vi "Process.vi"(8 "error in":errorcluster, 11 "DisplayWaveforms":refnum<class "DisplayWaveforms.lvclass">) -> (0 "error out":errorcluster, 3 "DisplayWaveforms out":refnum<class "DisplayWaveforms.lvclass">)   [LabVIEW 2020, in "DisplayWaveform.lvlib" / "DisplayWaveforms.lvclass"]
doc: "Displays all the waveforms using charts."
uses:
  DisplayWaveforms.lvclass
  C:/Program Files (x86)/National Instruments/LabVIEW 2020/vi.lib/JKI/JKI SMO/SMO/SMO.lvclass
  C:/Program Files (x86)/National Instruments/LabVIEW 2020/vi.lib/JKI/JKI SMO/SMO.UI/SMO.UI.lvclass
  <vilib>/JKI/JKI SMO/SMO/Typedefs/Parent Call--Enum.ctl
  PumpMeas/TypeDefs/ChartParamsCluster.ctl
  PumpMeas/TypeDefs/NI9205offset.ctl
  PumpMeas/TypeDefs/NI9205multiplier.ctl
  PumpMeas/TypeDefs/NI9208offset.ctl
  PumpMeas/TypeDefs/NI9208multiplier.ctl
  DisplayWaveforms.lvclass/DisplayWaveforms.ctl
  <vilib>/JKI/JKI SMO/SMO.UI/SMO.UI.lvclass
  <vilib>/JKI/JKI SMO/SMO/SMO.lvclass
panel:
  out "<TBD>":dbl[][](graph)
  out "<TBD>":dbl[][](graph)
  out "NI9208 Signals":dbl[][](graph)
  out "NI 9205 Signals":dbl[][](graph)
  out "NI9205 Signals":dbl[][](graph)
  in  "------------- Registered Events -------------":bool
  in  "------------- Public API -------------":bool
  # "For instructions on how to use the JKI State Machine Objects, examples and video tutorials, visit:\nhttp://jki.net/state-machine-objects/\n\nJKI State Machine Objects™\nhttp://jki.net/state-machine-objects/\nCopyright (C) 2005-2015, JKI <info@jki.net>\nALL RIGHTS RESERVED"
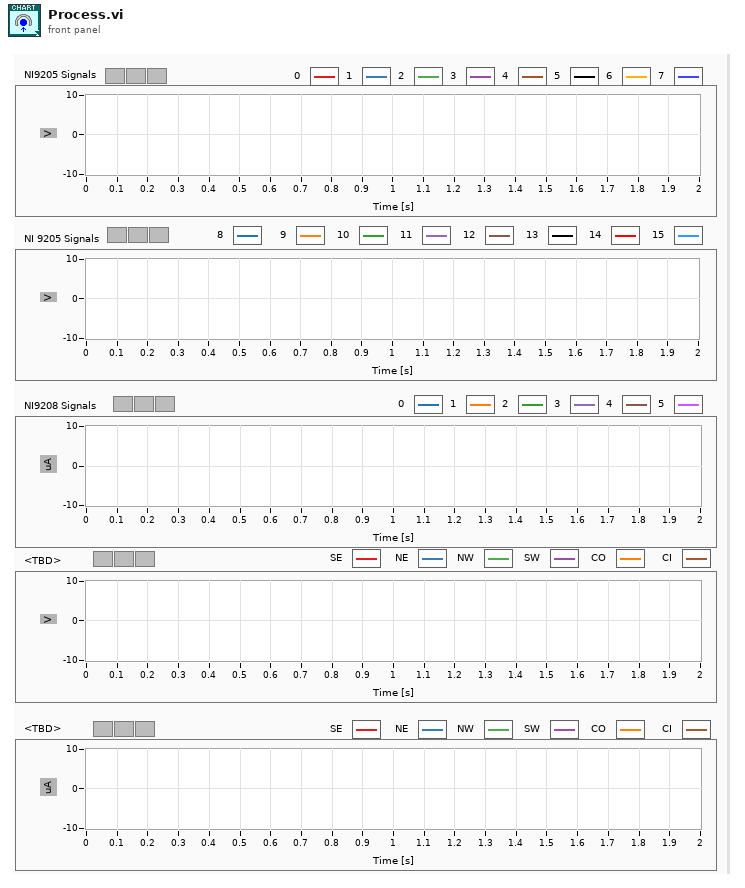
[diagram p1: front panel]
types:
  T1 = typedef "SMO.lvclass/Parent Call--Enum.ctl" = enum16{"Allows parent to run", "Does not request parent to run"}
  T2 = enum32{"invalid app kind", "Development System", "Run Time System", "Student Edition", "Embedded LabVIEW", "Evaluation", "Custom"}
  T3 = enum32{"Invalid", "Standard", "Closed", "Hidden", "Minimized", "Maximized"}
  T4 = typedef "ChartParamsCluster.ctl" = cluster{"Chart ScaleMultipliers":cluster{"WF Xscale Multiplier":dbl, "WF Yscale Multiplier":dbl[]}, "NI9205 Offset":T5, "NI9205 Multipliers":T6, "NI9208 Offset":T7, "NI9208 Multiplier":T8}
  T5 = typedef "NI9205offset.ctl" = cluster{"NI9205 Offset":dbl[]}
  T6 = typedef "NI9205multiplier.ctl" = cluster{"NI9205 Multiplier":dbl[]}
  T7 = typedef "NI9208offset.ctl" = cluster{"NI9208 Offset":dbl[]}
  T8 = typedef "NI9208multiplier.ctl" = cluster{"NI9208 Multiplier":dbl[]}
  T9 = cluster{"Core":cluster{"Current VI Reference":refnum<vi>, "Close Panel on Exit?":bool, "error":errorcluster}, "Self Reference":refnum<class "DisplayWaveforms.lvclass">, "bool":bool, "update chart?":bool, "ChartParams":T4, "Export Folder Path":path}
  T10 = cluster{"Current VI Reference":refnum<vi>, "Close Panel on Exit?":bool, "error":errorcluster}
  T11 = typedef "SMO.lvclass/Protected Events.ctl" = cluster{"StopProcesses":refnum<user-event>, "AbortProcesses":refnum<user-event>, "Config Changed":refnum<user-event>, "Dependency":refnum<user-event>}
  T12 = typedef "DisplayWaveform.lvlib/DisplayWaveforms.lvclass/ProtectedEvents--Cluster.ctl" = cluster{"Clear Chart":refnum<user-event>, "Pause Chart":refnum<user-event>, "Update Chart":refnum<user-event>, "Export Chart":refnum<user-event>, "Set ChartParams":refnum<user-event>}
  T13 = typedef "DisplayWaveform.lvlib/DisplayWaveforms.lvclass/Dependencies--Cluster.ctl" = cluster{"New Value":refnum<user-event>}
  T14 = typedef "imagedata.ctl" = cluster{"image type":i32, "image depth":i32, "image":u8[], "mask":u8[], "colors":u32[], "Rectangle":cluster{"left":i16, "top":i16, "right":i16, "bottom":i16}}
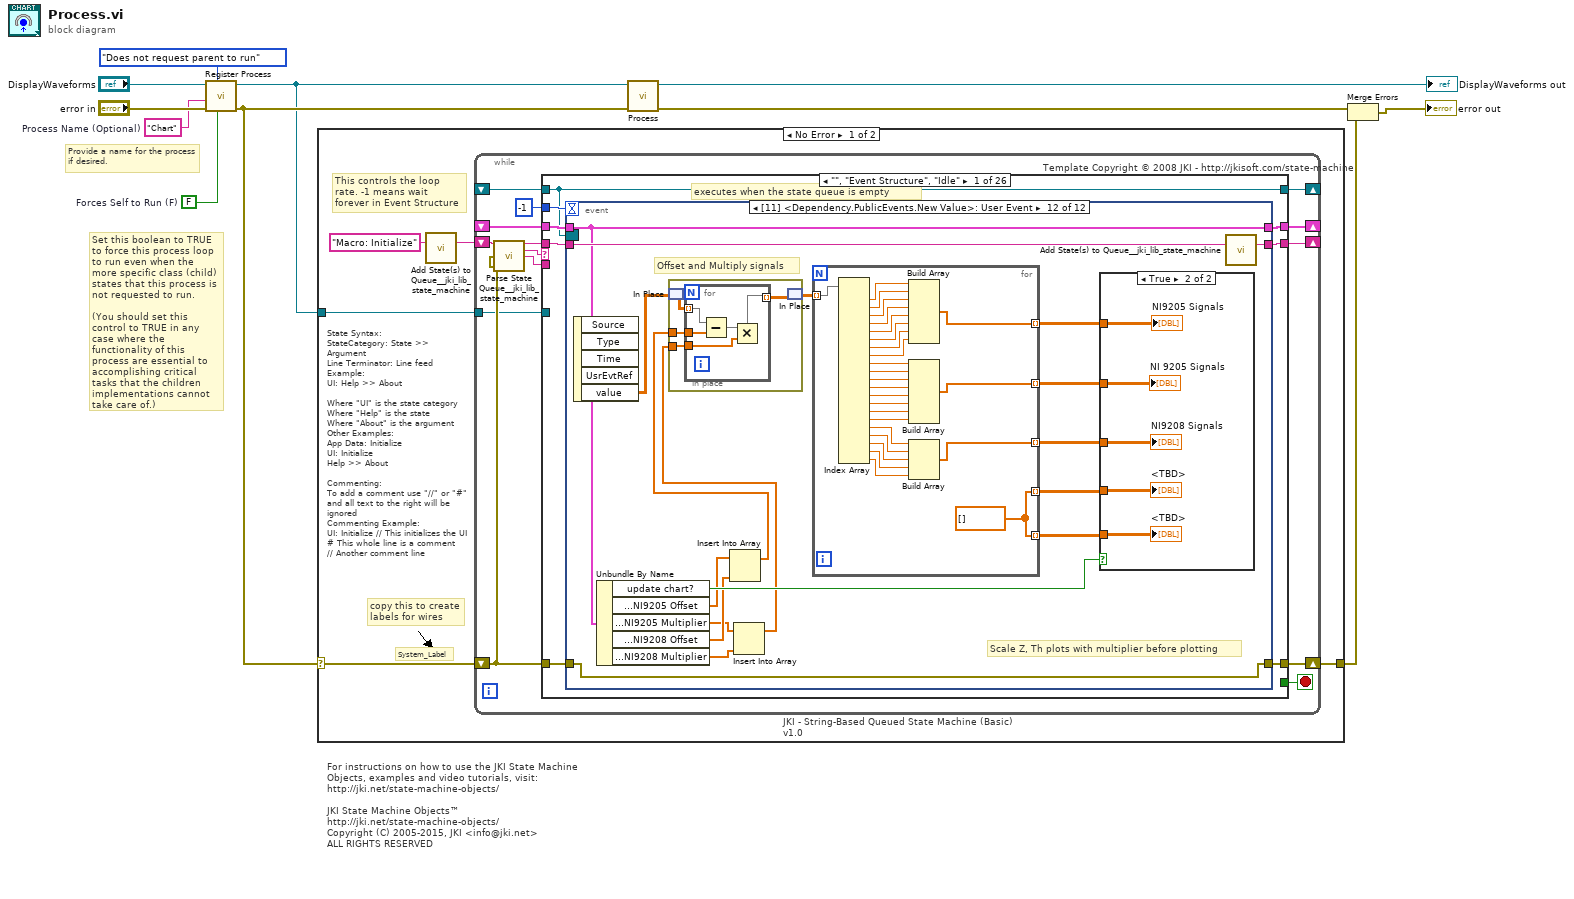
[diagram p0: block diagram]
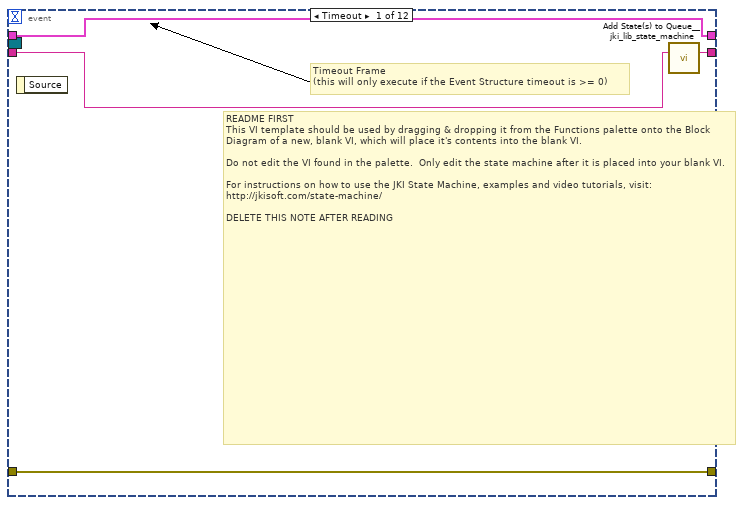
[diagram p2: hidden frame]
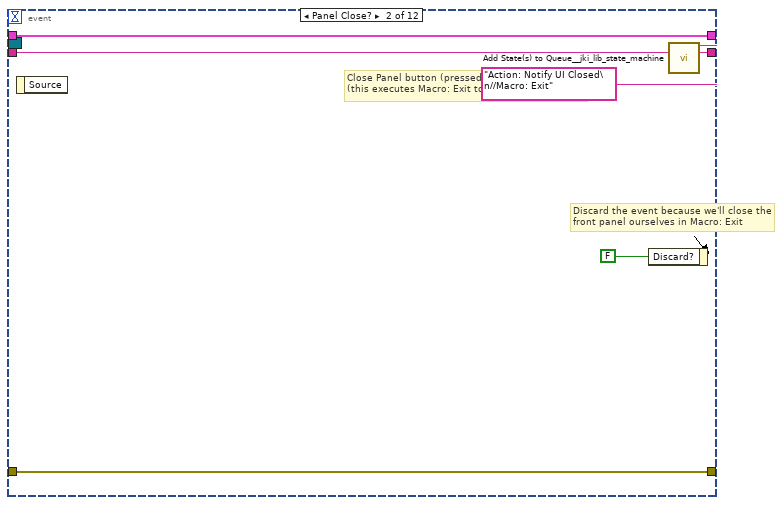
[diagram p3: hidden frame]
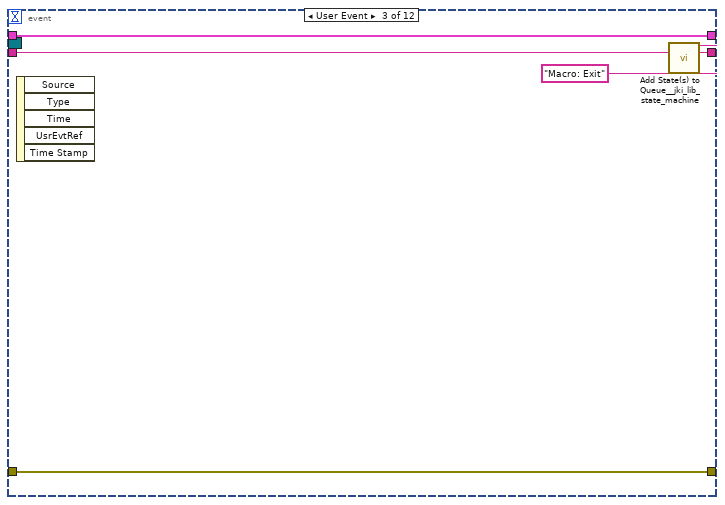
[diagram p4: hidden frame]
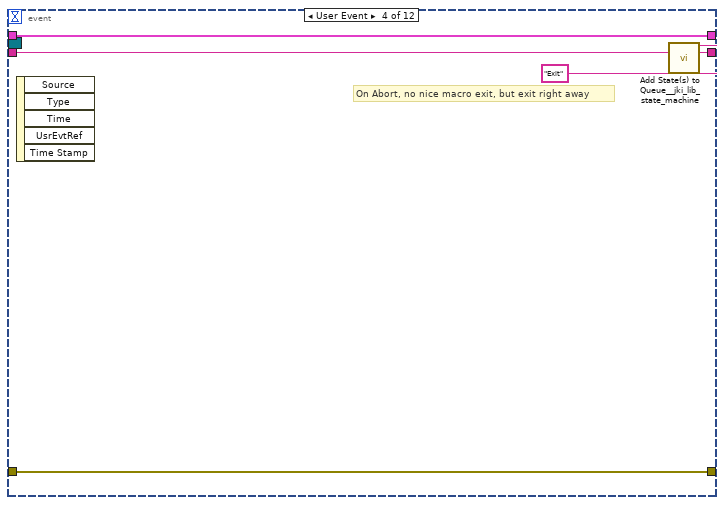
[diagram p5: hidden frame]
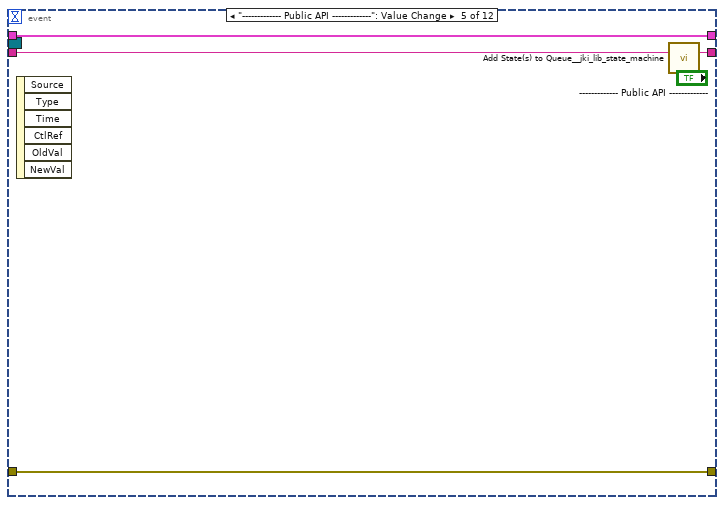
[diagram p6: hidden frame]
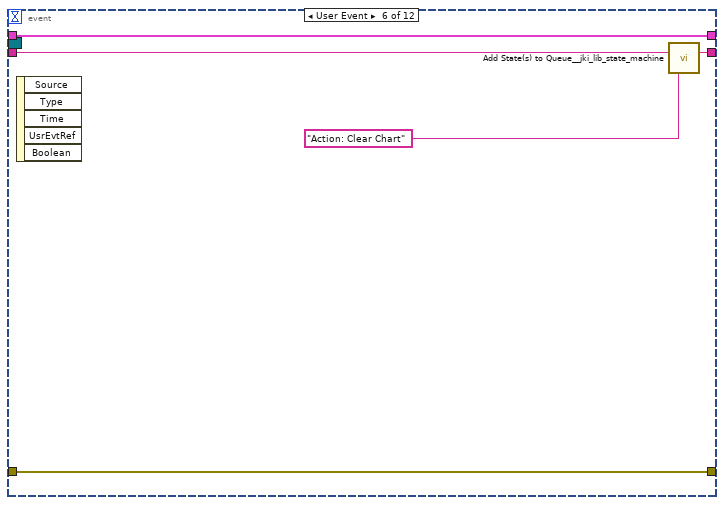
[diagram p7: hidden frame]
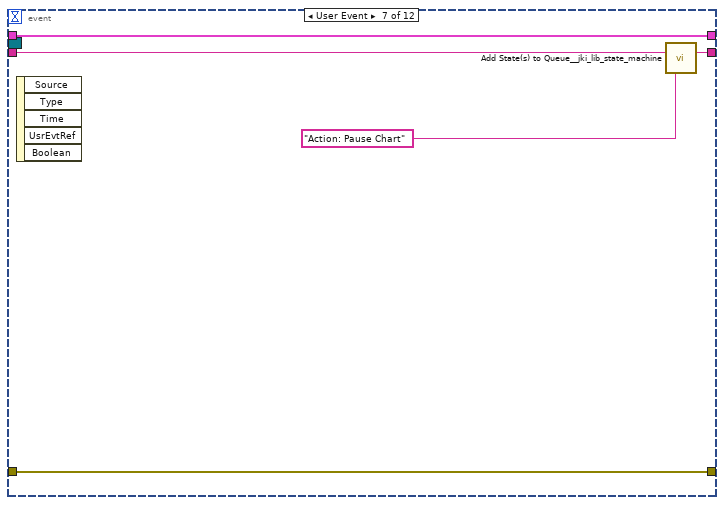
[diagram p8: hidden frame]
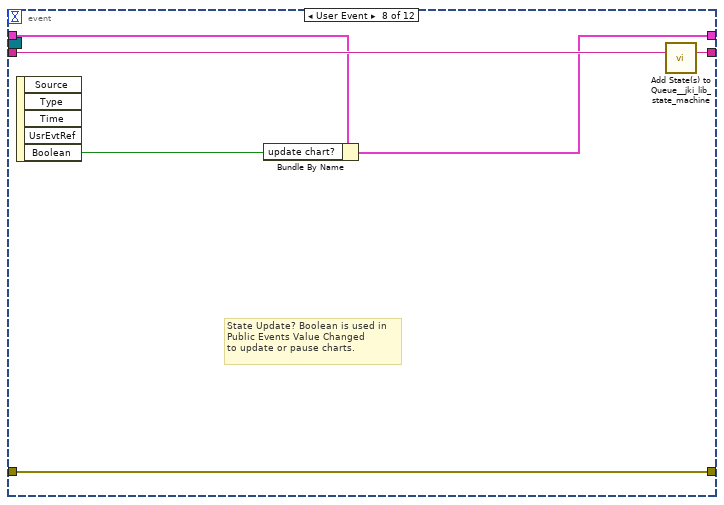
[diagram p9: hidden frame]
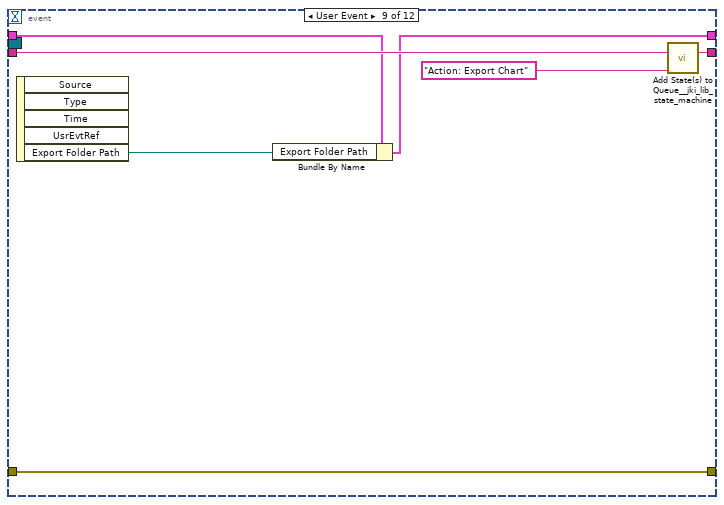
[diagram p10: hidden frame]
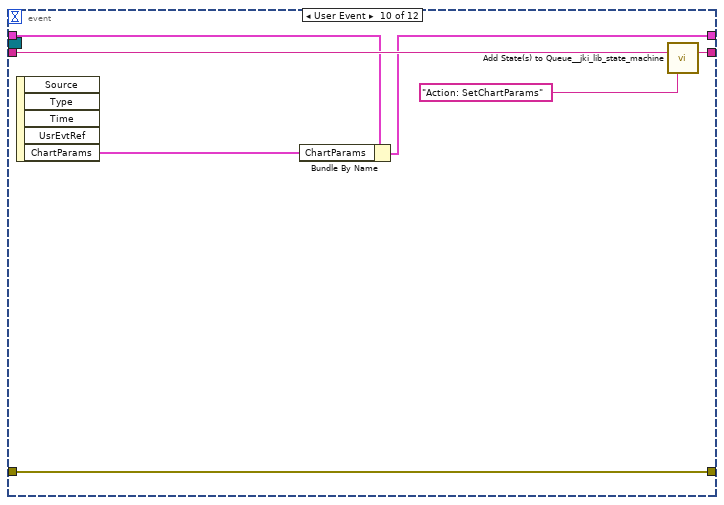
[diagram p11: hidden frame]
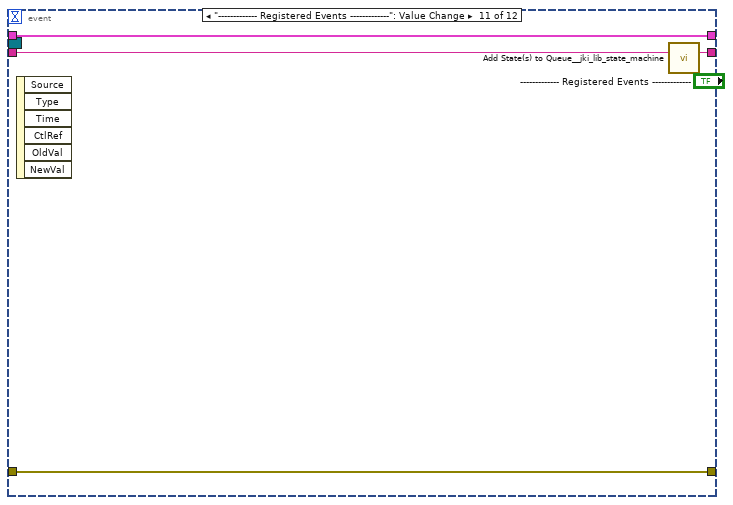
[diagram p12: hidden frame]
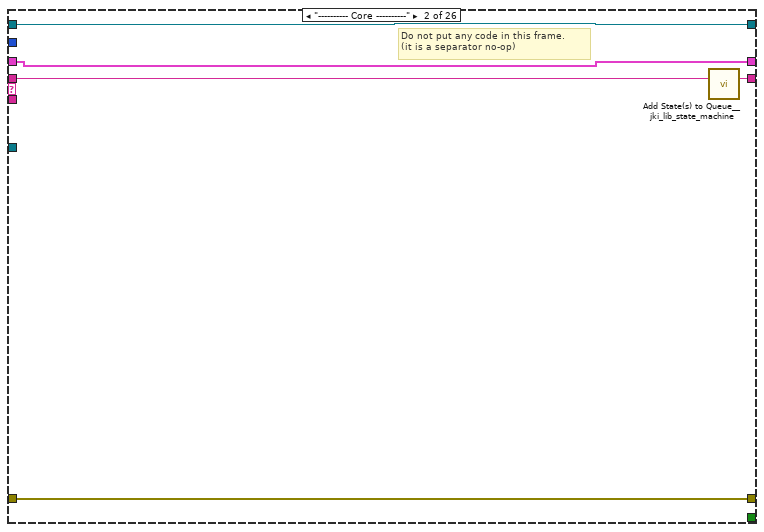
[diagram p14: hidden frame]
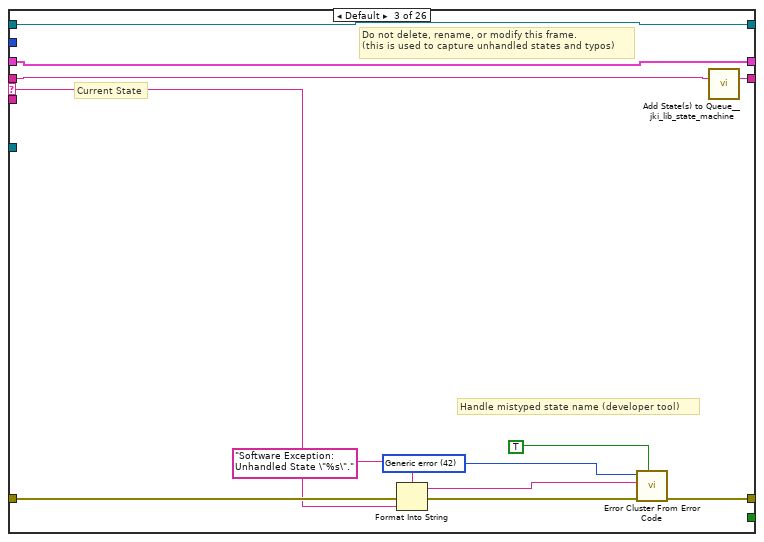
[diagram p15: hidden frame]
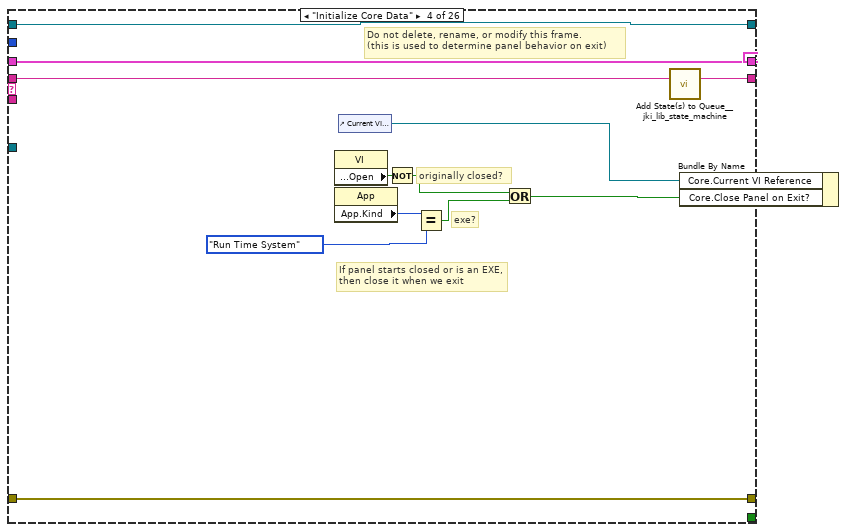
[diagram p16: hidden frame]
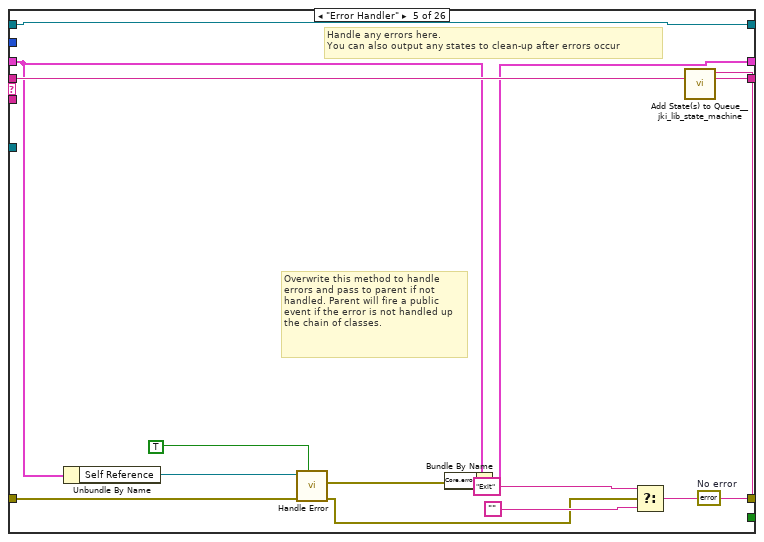
[diagram p17: hidden frame]
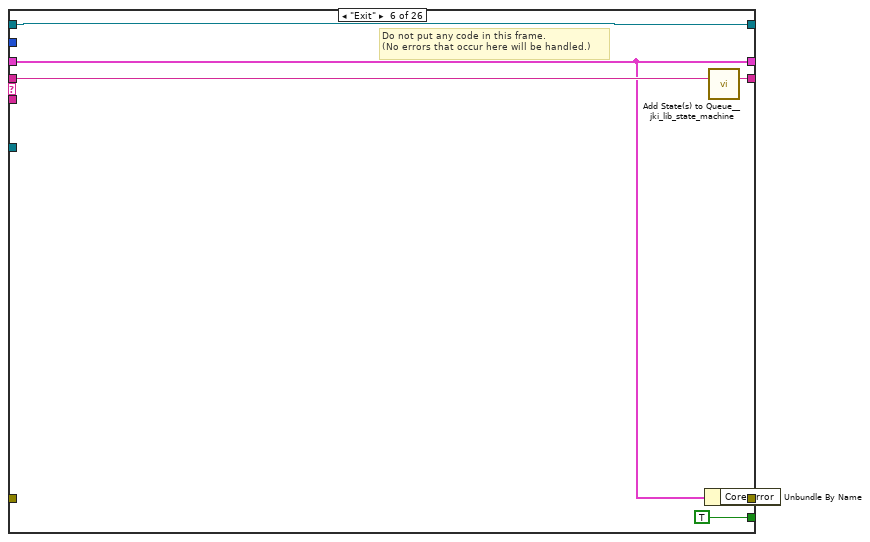
[diagram p18: hidden frame]
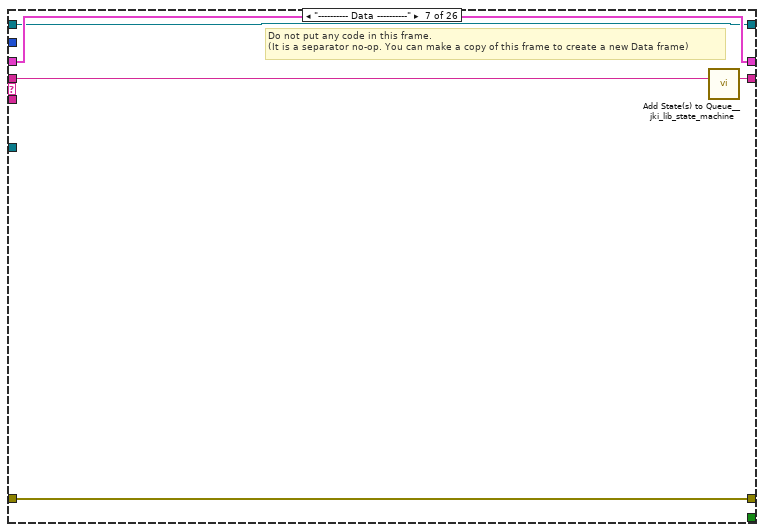
[diagram p19: hidden frame]
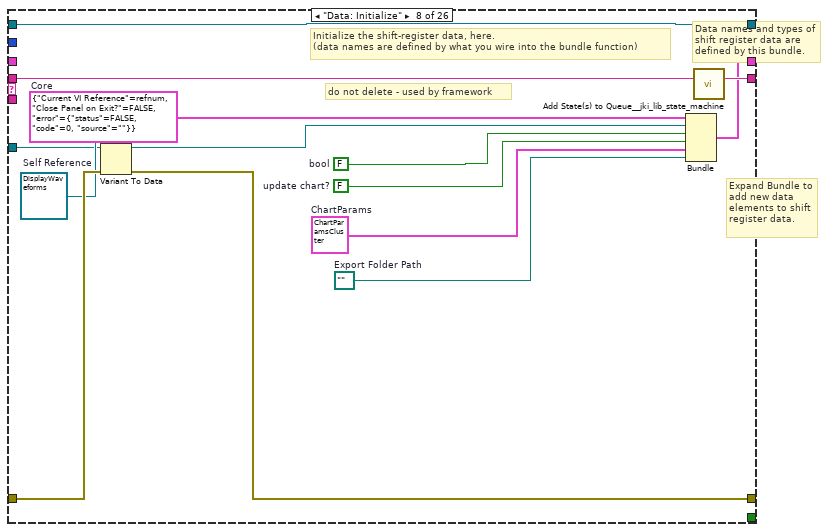
[diagram p20: hidden frame]
diagram:
  w2 = FALSE  # Forces Self to Run (F)
  w1 = "Chart"  # Process Name (Optional)
  # "Provide a name for the process\nif desired."
  # "Set this boolean to TRUE to force this process loop to run even when the more specific class (child) states that this process is not requested to run.\n\n(You should set this control to TRUE in any case where the functionality of this process are essential to accomplishing critical tasks that the children implementations cannot take care of.)"
  # "For instructions on how to use the JKI State Machine Objects, examples and video tutorials, visit:\nhttp://jki.net/state-machine-objects/\n\nJKI State Machine Objects™\nhttp://jki.net/state-machine-objects/\nCopyright (C) 2005-2015, JKI <info@jki.net>\nALL RIGHTS RESERVED"
  n1 = call <vilib>:"Register Process.vi"("Forces Self to Run (F)"=w2, "Parent Call"=Parent_Call--Enum."Does not request parent to run", "error in (no error)"="error in", "Process Name (optional)"=w1, "SMO"="DisplayWaveforms") -> ("error out"=w8:errorcluster, "SMO out"=w7:refnum<class "DisplayWaveforms.lvclass">)  [unwired: 5 in]
  n2 = case shown="No Error" w8 {
    selector: w8 -> [w13 w422]
    tunnel: w7 -> [w14 _]
    tunnel: [w12 w422] -> w4
    frame No Error {
      # "State Syntax:\nStateCategory: State >> Argument\nLine Terminator: Line feed\nExample:\nUI: Help >> About\n\nWhere \"UI\" is the state category\nWhere \"Help\" is the state\nWhere \"About\" is the argument\nOther Examples:\nApp Data: Initialize\nUI: Initialize\nHelp >> About\n\nCommenting:\nTo add a comment use \"//\" or \"#\" and all text to the right will be ignored\nCommenting Example:\nUI: Initialize // This initializes the UI\n# This whole line is a comment\n// Another comment line"
      # "copy this to create labels for wires"
      # "This controls the loop rate. -1 means wait forever in Event Structure"
      # "System_Label"
      n3 = call <vilib>:"Add State(s) to Queue__jki_lib_state_machine.vi"("State(s) in (\"\")"="Macro: Initialize") -> ("States Out"=w16:string)  [unwired: 14 in]
      n4 = while "JKI - String-Based Queued State Machine (Basic) v1.0" {
        shift-right: [w23] -> _
        shift-left: _ -> [w22]
        shift-right: [w26] -> w12
        shift-left: w13 -> [w20]
        shift-right: [w25] -> _
        shift-left: w16 -> [w27]
        tunnel: w14 -> [w19]
        shift-right: [w18] -> _
        shift-left: _ -> [w17]
        stop <- w24 stop-if-true
        # "Template Copyright © 2008 JKI - http://jkisoft.com/state-machine"
        n5 = call <vilib>:"Parse State Queue__jki_lib_state_machine.vi"("State Queue"=w27, "Error In (no error)"=w20) -> ("Remaining States"=w29:string, "Current State"=w30:string, "Arguments"=w28:string)  [unwired: 11 in]
        n6 = case shown="\"\", \"Event Structure\", \"Idle\"" w30 {
          selector: w30 -> [_ _ w161 _ _ _ _ _ _ _ _ _ _ _ _ _ _ _ _ _ _ _ _ _ _ _]
          tunnel: w29 -> [w38 w159 w165 w184 w198 w204 w209 w223 w230 w235 w248 w255 w271 w303 w312 w326 w331 w342 w347 w365 w377 w382 w389 w405 w414 w421]
          tunnel: w28 -> [_ _ _ _ _ _ _ _ _ _ _ w249 w265 _ _ _ _ _ _ _ _ _ _ _ _ _]
          tunnel: w22 -> [w36 w156 w163 w175 w187 w200 w206 _ w225 w232 w244 w253 w267 w300 w308 w317 w328 w339 w344 w363 w375 w380 w386 w402 w411 w417]
          tunnel: [w35 w157 w167 w181 w189 w199 w207 w218 w226 w233 w246 w250 w268 w301 w310 w324 w329 w333 w345 w360 w373 w378 w384 w392 w409 w415] -> w26
          tunnel: w20 -> [w34 w157 w166 w181 w194 _ w207 w219 w227 w233 w246 w251 w269 w301 w310 w324 w329 w334 w345 w356 w373 w378 w385 w401 w410 w416]
          tunnel: [w37 w158 w164 w183 w197 w203 w208 w222 w229 w234 w247 w254 w270 w302 w311 w325 w330 w341 w346 w364 w376 w381 w388 w404 w413 w420] -> w25
          tunnel: [_ _ _ _ _ TRUE _ _ _ _ _ _ _ _ _ _ _ _ _ _ _ _ _ _ _ _] -> w24
          tunnel: [w33 w156 w163 w182 w186 w200 w206 w221 w225 w232 w243 w253 w267 w300 w308 w317 w328 w339 w344 w363 w375 w380 w386 w402 w411 w417] -> w23
          tunnel: -1 ("Timeout") -> [w32 _ _ _ _ _ _ _ _ _ _ _ _ _ _ _ _ _ _ _ _ _ _ _ _ _]
          tunnel: w19 -> [_ _ _ _ _ _ _ w216 _ _ _ _ _ _ _ _ _ _ _ _ _ _ _ _ _ _]
          tunnel: [w31 w155 w160 w172 w196 w201 w205 w214 w224 w231 w245 w252 w264 w299 w309 w318 w327 w340 w343 w362 w374 w379 w387 w403 w412 w419] -> w18
          tunnel: w17 -> [w31 w155 w160 w172 w196 w201 w205 w214 w224 w231 w245 w252 w264 w299 w309 w318 w327 w340 w343 _ w374 w379 w387 w403 w412 w419]
          frame "", "Event Structure", "Idle" {
            # "executes when the state queue is empty"
            n7 = event shown="[11] <Dependency.PublicEvents.New Value>: User Event" {
              selector: w31 -> [_ _ _ _ _ _ _ _ _ _ _ _]
              dyn-events: _ -> [_ _ _ _ _ _ _ _ _ _ _ _]
              timeout: w32 -> [_ _ _ _ _ _ _ _ _ _ _ _]
              tunnel: w38 -> [w42 w48 w53 w58 w62 w67 w71 w78 w84 w91 w96 w114]
              tunnel: [w41 w47 w52 w57 w61 w66 w69 w77 w83 w90 w95 w113] -> w37
              tunnel: w36 -> [w39 w44 w50 w55 w59 w64 w70 w75 w81 w88 w93 w108]
              tunnel: [w40 w43 w51 w56 w60 w65 w68 w76 w82 w89 w94 w112] -> w35
              tunnel: w34 -> [w40 w43 w51 w56 w60 w65 w68 w76 w82 w89 w94 w112]
              tunnel: [w39 w44 w50 w55 w59 w64 w70 w73 w79 w86 w93 w108] -> w33
              event Timeout {
                # "README FIRST\nThis VI template should be used by dragging & dropping it from the Functions palette onto the Block Diagram of a new, blank VI, which will place it's contents into the blank VI.\n\nDo not edit the VI found in the palette.  Only edit the state machine after it is placed into your blank VI.\n\nFor instructions on how to use the JKI State Machine, examples and video tutorials, visit:\nhttp://jkisoft.com/state-machine/\n\nDELETE THIS NOTE AFTER READING"
                # "Timeout Frame\n(this will only execute if the Event Structure timeout is >= 0)"
                n8 = event-data() -> ()  [unwired: 1 in, 1 out]
                n9 = call <vilib>:"Add State(s) to Queue__jki_lib_state_machine.vi"("State(s) in (\"\")"=w42) -> ("States Out"=w41:string)  [unwired: 14 in]
              }
              event Panel Close? {
                # "Discard the event because we'll close the front panel ourselves in Macro: Exit"
                # "Close Panel button (pressed) Event\n(this executes Macro: Exit to terminate the VI)"
                n10 = event-data() -> ()  [unwired: 1 in, 1 out]
                n11 = event-data("Discard?"=FALSE) -> ()  [unwired: 1 in, 1 out]
                n12 = call <vilib>:"Add State(s) to Queue__jki_lib_state_machine.vi"("State(s) in Front (\"\")"="Action: Notify UI Closed\n//Macro: Exit", "State(s) in (\"\")"=w48) -> ("States Out"=w47:string)  [unwired: 13 in]
              }
              event User Event {
                n13 = event-data() -> ()  [unwired: 1 in, 5 out]
                n14 = call <vilib>:"Add State(s) to Queue__jki_lib_state_machine.vi"("State(s) in Front (\"\")"="Macro: Exit", "State(s) in (\"\")"=w53) -> ("States Out"=w52:string)  [unwired: 13 in]
              }
              event User Event {
                # "On Abort, no nice macro exit, but exit right away"
                n15 = event-data() -> ()  [unwired: 1 in, 5 out]
                n16 = call <vilib>:"Add State(s) to Queue__jki_lib_state_machine.vi"("State(s) in Front (\"\")"="Exit", "State(s) in (\"\")"=w58) -> ("States Out"=w57:string)  [unwired: 13 in]
              }
              event "------------- Public API -------------": Value Change {
                n17 = event-data() -> ()  [unwired: 1 in, 6 out]
                n18 = call <vilib>:"Add State(s) to Queue__jki_lib_state_machine.vi"("State(s) in (\"\")"=w62) -> ("States Out"=w61:string)  [unwired: 14 in]
              }
              event User Event {
                n19 = event-data() -> ()  [unwired: 1 in, 5 out]
                n20 = call <vilib>:"Add State(s) to Queue__jki_lib_state_machine.vi"("State(s) in Front (\"\")"="Action: Clear Chart", "State(s) in (\"\")"=w67) -> ("States Out"=w66:string)  [unwired: 13 in]
              }
              event User Event {
                n21 = event-data() -> ()  [unwired: 1 in, 5 out]
                n22 = call <vilib>:"Add State(s) to Queue__jki_lib_state_machine.vi"("State(s) in Front (\"\")"="Action: Pause Chart", "State(s) in (\"\")"=w71) -> ("States Out"=w69:string)  [unwired: 13 in]
              }
              event User Event {
                # "State Update? Boolean is used in \nPublic Events Value Changed \nto update or pause charts."
                n23 = event-data() -> ("Boolean"=w74:bool)  [unwired: 1 in, 4 out]
                n24 = Bundle By Name(cluster=w75, "update chart?"=w74) -> (w73:T9)
                n25 = call <vilib>:"Add State(s) to Queue__jki_lib_state_machine.vi"("State(s) in (\"\")"=w78) -> ("States Out"=w77:string)  [unwired: 14 in]
              }
              event User Event {
                n26 = event-data() -> ("Export Folder Path"=w80:path)  [unwired: 1 in, 4 out]
                n27 = Bundle By Name(cluster=w81, "Export Folder Path"=w80) -> (w79:T9)
                n28 = call <vilib>:"Add State(s) to Queue__jki_lib_state_machine.vi"("State(s) in Front (\"\")"="Action: Export Chart", "State(s) in (\"\")"=w84) -> ("States Out"=w83:string)  [unwired: 13 in]
              }
              event User Event {
                n29 = event-data() -> ("ChartParams"=w87:T4)  [unwired: 1 in, 4 out]
                n30 = Bundle By Name(cluster=w88, "ChartParams"=w87) -> (w86:T9)
                n31 = call <vilib>:"Add State(s) to Queue__jki_lib_state_machine.vi"("State(s) in Front (\"\")"="Action: SetChartParams", "State(s) in (\"\")"=w91) -> ("States Out"=w90:string)  [unwired: 13 in]
              }
              event "------------- Registered Events -------------": Value Change {
                n32 = event-data() -> ()  [unwired: 1 in, 6 out]
                n33 = call <vilib>:"Add State(s) to Queue__jki_lib_state_machine.vi"("State(s) in (\"\")"=w96) -> ("States Out"=w95:string)  [unwired: 14 in]
              }
              event User Event {
                # "Offset and Multiply signals"
                # "Scale Z, Th plots with multiplier before plotting"
                n34 = event-data() -> ("value"=w106:dbl[][])  [unwired: 1 in, 4 out]
                n35 = Unbundle By Name(w108) -> ("update chart?"=w107:bool, "ChartParams.NI9205 Offset.NI9205 Offset"=w104:dbl[], "ChartParams.NI9205 Multipliers.NI9205 Multiplier"=w100:dbl[], "ChartParams.NI9208 Offset.NI9208 Offset"=w103:dbl[], "ChartParams.NI9208 Multiplier.NI9208 Multiplier"=w99:dbl[])
                n36 = Insert Into Array(array=w104, new element=w103) -> (w102:dbl[])  [unwired: 1 in]
                n37 = Insert Into Array(array=w100, new element=w99) -> (w101:dbl[])  [unwired: 1 in]
                n38 = in-place {
                  in-place-border: w102 -> [w117]
                  in-place-border: w101 -> [w116]
                  n39 = in-place-match #1(w106) -> (w118:dbl[][])
                  n40 = for {
                    tunnel: w118 -> [w122] mode=indexing
                    tunnel: [w123] -> w115 mode=indexing
                    tunnel: w117 -> [w121]
                    tunnel: w116 -> [w119]
                    n41 = Subtract(x=w122, y=w121) -> (x-y=w120:dbl[])
                    n42 = Multiply(x=w120, y=w119) -> (x*y=w123:dbl[])
                  }
                  n43 = in-place-match #1(w115) -> (w105:dbl[][])
                }
                n44 = for {
                  tunnel: w105 -> [w154] mode=indexing
                  tunnel: [w153] -> w111 mode=indexing
                  tunnel: [w131] -> w110 mode=indexing
                  tunnel: [w130] -> w109 mode=indexing
                  tunnel: [w129] -> w98 mode=indexing
                  tunnel: [w129] -> w97 mode=indexing
                  w129 = dbl[] [] ("appended array")
                  n45 = Index Array(array=w154) -> (element #1=w152:dbl, element #2=w151:dbl, element #3=w150:dbl, element #4=w149:dbl, element #5=w148:dbl, element #6=w147:dbl, element #7=w146:dbl, element #8=w145:dbl, element #9=w144:dbl, element #10=w143:dbl, element #11=w142:dbl, element #12=w141:dbl, element #13=w140:dbl, element #14=w139:dbl, element #15=w138:dbl, element #16=w137:dbl, element #17=w136:dbl, element #18=w135:dbl, element #19=w134:dbl, element #20=w133:dbl, element #21=w132:dbl)  [unwired: 21 in]
                  n46 = Build Array(w152, w151, w150, w149, w148, w147, w146, w145) -> (w153:dbl[])
                  n47 = Build Array(w144, w143, w142, w141, w140, w139, w138, w137) -> (w131:dbl[])
                  n48 = Build Array(w136, w135, w134, w133, w132) -> (w130:dbl[])
                }
                n49 = case shown="True" w107 {
                  tunnel: w111 -> [_ w128]
                  tunnel: w110 -> [_ w126]
                  tunnel: w109 -> [_ w127]
                  tunnel: w98 -> [_ w125]
                  tunnel: w97 -> [_ w124]
                  frame False {
                  }
                  frame True {
                    "NI 9205 Signals" <- w126
                    "NI9205 Signals" <- w128
                    "<TBD>" <- w124
                    "<TBD>" <- w125
                    "NI9208 Signals" <- w127
                  }
                }
                n50 = call <vilib>:"Add State(s) to Queue__jki_lib_state_machine.vi"("State(s) in (\"\")"=w114) -> ("States Out"=w113:string)  [unwired: 14 in]
              }
            }
          }
          frame "---------- Core ----------" {
            # "Do not put any code in this frame.\n(it is a separator no-op)"
            n51 = call <vilib>:"Add State(s) to Queue__jki_lib_state_machine.vi"("State(s) in (\"\")"=w159) -> ("States Out"=w158:string)  [unwired: 14 in]
          }
          frame Default {
            w170 = 42 items=["No error", "Argument error", "Memory is full", "Out of zone", "End of file", "File already open", "Generic file I/O error", "File not found", "File permission error", "Disk is full", "Duplicate path", "Too many files open", "System feature not enabled", "Resource file not found", "Cannot add resource", "Resource not found", "Image not found", "Image memory error", "Pen does not exist", "Config type invalid", "Config token not found", "Config parse error", "Config memory error", "Bad external code format", "Bad external code offset", "External code not present", "Null window", "Destroy window error", "Null menu", "Print aborted", "Bad print record", "Print driver error", "Windows error during printing", "Memory error during printing", "Print dialog error", "Generic print error", "Invalid device refnum", "Device not found", "Device parameter error", "Device unit error", "Cannot open device", "Device call aborted", "Generic error", "Cancelled by user", "Object ID too low", "Object ID too high", "Object not in heap", "Unknown heap", "Unknown object (invalid DefProc)", "Unknown object (DefProc not in table)", "Message out of range", "Invalid (null) method", "Unknown message", "Manager call not supported", "Bad address", "Network operation in progress", "Network operation timed out", "Connection is busy", "Network attribute not supported", "Network error", "Address in use", "System out of memory", "Connection aborted", "Connection refused", "Not connected", "Already connected", "Connection closed", "Initialization error (interapplication manager)", "Bad occurrence", "Wait on unbound occurrence handler", "Occurrence queue overflow", "Datalog type conflict", "Unused", "Unrecognized type (interapplication manager)", "Memory corrupt", "Failed to make temporary DLL", "Old CIN version", "Drag socket not found", "Failed to load drop-object", "Failed to register OLE object", "Failed to release OLE object", "Format specifier type mismatch", "Unknown format specifier", "Too few format specifiers", "Too many format specifiers", "Scan failed", "Newer CIN version", "Error converting to variant", "Runtime menu error", "Password tampered", "Variant attribute not found", "Incompatible variant data type", "Event data is not available", "Event Store is not present", "Occurrence is not found", "Event Queue is not created", "Event info is not available", "Refnum passed is NULL", "Error retrieving Class GUID", "Error retrieving CoClass GUID", "Error retrieving TypeLib GUID.", "Bad built application magic bytes.", "Specific driver is different from the specific driver associated with the Logical Name.", "There is no session opened to the class driver.", "Max Error", "MAX - Error with config objects", "MAX - Error loading configuration", "MAX - Group not supported"]
            # "Current State"
            # "Do not delete, rename, or modify this frame.\n(this is used to capture unhandled states and typos)"
            # "Handle mistyped state name (developer tool)"
            n52 = Format Into String(format string="Software Exception: Unhandled State \"%s\"." ("message"), error in=w166, w161) -> (resulting string=w169:string, error out=w168:errorcluster)  [unwired: 1 in]
            n53 = call <vilib>:"Error Cluster From Error Code.vi"("show call chain? (False)"=TRUE, "error in (no error)"=w168, "error message (\"\")"=w169, "error code (0)"=w170) -> ("error out"=w167:errorcluster)  [unwired: 5 in]
            n54 = call <vilib>:"Add State(s) to Queue__jki_lib_state_machine.vi"("State(s) in (\"\")"=w165) -> ("States Out"=w164:string)  [unwired: 14 in]
          }
          frame "Initialize Core Data" {
            # "Do not delete, rename, or modify this frame.\n(this is used to determine panel behavior on exit)"
            # "originally closed?"
            # "exe?"
            # "If panel starts closed or is an EXE, then close it when we exit"
            n55 = property class="VI"() -> ("Front Panel.Open"=w180:bool)  [unwired: 2 in, 2 out]
            n56 = property class="App"() -> ("App.Kind"=w179:T2)  [unwired: 2 in, 2 out]
            n57 = control-ref of="Current VI Reference"() -> (w173:refnum<vi>)
            n58 = Not(x=w180) -> (.not. x?=w177:bool)
            n59 = Equal?(x=w179, y=T2."Run Time System" ("Application:Kind")) -> (x = y?=w176:bool)
            n60 = Or(x=w177, y=w176) -> (x .or. y?=w174:bool)
            n61 = call <vilib>:"Add State(s) to Queue__jki_lib_state_machine.vi"("State(s) in (\"\")"=w184) -> ("States Out"=w183:string)  [unwired: 14 in]
            n62 = Bundle By Name(cluster=w175, "Core.Current VI Reference"=w173, "Core.Close Panel on Exit?"=w174) -> (w182:T9)
          }
          frame "Error Handler" {
            w189 = errorcluster {"status"=FALSE, "code"=0, "source"=""}  # No error
            # "Overwrite this method to handle errors and pass to parent if not handled. Parent will fire a public event if the error is not handled up the chain of classes."
            # "Handle any errors here.\nYou can also output any states to clean-up after errors occur"
            n63 = Unbundle By Name(w187) -> ("Self Reference"=w195:refnum<class "DisplayWaveforms.lvclass">)
            n64 = call-dynamic "Handle Error.vi"("Stop on Unhandled Error (T)"=TRUE, "error in"=w194, "SMO"=w195) -> ("handling error"=w190:errorcluster, "Unhandled error"=w188:errorcluster)  [unwired: 6 in, 1 out]
            n65 = Bundle By Name(cluster=w187, "Core.error"=w188) -> (w186:T9)
            n66 = Select(t="Exit", s=w190, f="") -> (s? t:f=w191:string)
            n67 = call <vilib>:"Add State(s) to Queue__jki_lib_state_machine.vi"("State(s) in Front (\"\")"=w191, "State(s) in (\"\")"=w198) -> ("States Out"=w197:string)  [unwired: 13 in]
          }
          frame "Exit" {
            # "Do not put any code in this frame.\n(No errors that occur here will be handled.)"
            n68 = Unbundle By Name(w200) -> ("Core.error"=w199:errorcluster)
            n69 = call <vilib>:"Add State(s) to Queue__jki_lib_state_machine.vi"("State(s) in (\"\")"=w204) -> ("States Out"=w203:string)  [unwired: 14 in]
          }
          frame "---------- Data ----------" {
            # "Do not put any code in this frame.\n(It is a separator no-op. You can make a copy of this frame to create a new Data frame)"
            n70 = call <vilib>:"Add State(s) to Queue__jki_lib_state_machine.vi"("State(s) in (\"\")"=w209) -> ("States Out"=w208:string)  [unwired: 14 in]
          }
          frame "Data: Initialize" {
            w210 = path ""  # Export Folder Path
            w211 = T4 {"Chart ScaleMultipliers"={"WF Xscale Multiplier"=1000.0, "WF Yscale Multiplier"=[]}, "NI9205 Offset"={"NI9205 Offset"=[]}, "NI9205 Multipliers"={"NI9205 Multiplier"=[]}, "NI9208 Offset"={"NI9208 Offset"=[]}, "NI9208 Multiplier"={"NI9208 Multiplier"=[]}}  # ChartParams
            w212 = FALSE  # update chart?
            w213 = T10 {"Current VI Reference"=refnum, "Close Panel on Exit?"=FALSE, "error"={"status"=FALSE, "code"=0, "source"=""}}  # Core
            w217 = refnum<class "DisplayWaveforms.lvclass"> refnum  # Self Reference
            w220 = FALSE  # bool
            # "do not delete - used by framework"
            # "Expand Bundle to add new data elements to shift register data."
            # "Data names and types of shift register data are defined by this bundle."
            # "Initialize the shift-register data, here.\n(data names are defined by what you wire into the bundle function)"
            n71 = Variant To Data(error in=w219, type=w217, Variant=w216) -> (data=w215:refnum<class "DisplayWaveforms.lvclass">, error out=w218:errorcluster)
            n72 = Bundle("Core"=w213, "Self Reference"=w215, "bool"=w220, "update chart?"=w212, "ChartParams"=w211, "Export Folder Path"=w210) -> (w221:T9)  [unwired: 1 in]
            n73 = call <vilib>:"Add State(s) to Queue__jki_lib_state_machine.vi"("State(s) in (\"\")"=w223) -> ("States Out"=w222:string)  [unwired: 14 in]
          }
          frame "Data: Cleanup" {
            # "Cleanup any data and references, here.\n(this is called automatically, by the Macro: Exit)"
            n74 = Unbundle By Name(w225) -> ("Core.Current VI Reference"=w228:refnum<vi>)
            n75 = Close Reference(reference=w228, error in (no error)=w227) -> (error out=w226:errorcluster)
            n76 = call <vilib>:"Add State(s) to Queue__jki_lib_state_machine.vi"("State(s) in (\"\")"=w230) -> ("States Out"=w229:string)  [unwired: 14 in]
          }
          frame "---------- UI ----------" {
            # "Do not put any code in this frame.\n(It is a separator no-op. You can make a copy of this frame to create a new UI frame)"
            n77 = call <vilib>:"Add State(s) to Queue__jki_lib_state_machine.vi"("State(s) in (\"\")"=w235) -> ("States Out"=w234:string)  [unwired: 14 in]
          }
          frame "UI: Initialize" {
            # "Initialize the User Interface, here.\n(this is called automatically, by the Macro: Init)"
            n78 = control-ref of="NI9205 Signals"() -> (w240:refnum<vi>)
            n79 = control-ref of="NI 9205 Signals"() -> (w239:refnum<vi>)
            n80 = control-ref of="NI9208 Signals"() -> (w238:refnum<vi>)
            n81 = control-ref of="<TBD>"() -> (w237:refnum<vi>)
            n82 = control-ref of="<TBD>"() -> (w236:refnum<vi>)
            n83 = Unbundle By Name(w244) -> ("Self Reference"=w242:refnum<class "DisplayWaveforms.lvclass">)
            n84 = Bundle By Name(cluster=w242, "WFChart Refnum"=w240, "WFChart Refnum 2"=w239, "WFChart Refnum 3"=w238, "WFChart Refnum 4"=w237, "WFChart Refnum 5"=w236) -> (w241:refnum<class "DisplayWaveforms.lvclass">)
            n85 = Bundle By Name(cluster=w244, "Self Reference"=w241) -> (w243:T9)
            n86 = call <vilib>:"Add State(s) to Queue__jki_lib_state_machine.vi"("State(s) in (\"\")"=w248) -> ("States Out"=w247:string)  [unwired: 14 in]
          }
          frame "UI: Cursor Set" {
            # "Argument"
            # "Initialize the User Interface, here.\n(this is called automatically, by the Macro: Init)"
            n87 = disable-structure shown="Default" {
              disable-tunnel: w251 -> [w256 w259]
              disable-tunnel: [w256 w258] -> w250
              disable-tunnel: w249 -> [_ w257]
              frame condition #0 {
              }
              frame condition #1 (active) {
                n88 = case shown="\"Idle\", Default" w257 {
                  tunnel: w259 -> [w261 w263]
                  tunnel: [w260 w262] -> w258
                  frame "Idle", Default {
                    n89 = call <vilib>:"Unset Busy.vi"("error in (no error)"=w261) -> ("error out"=w260:errorcluster)  [unwired: 10 in]
                  }
                  frame "Busy" {
                    n90 = call <vilib>:"Set Busy.vi"("error in (no error)"=w263) -> ("error out"=w262:errorcluster)  [unwired: 9 in, 1 out]
                  }
                }
              }
            }
            n91 = call <vilib>:"Add State(s) to Queue__jki_lib_state_machine.vi"("State(s) in (\"\")"=w255) -> ("States Out"=w254:string)  [unwired: 14 in]
          }
          frame "UI: Front Panel State" {
            # "Argument"
            # "Set Front Panel Open or Closed\n(Usage: \"UI: Front Panel State >> Open|Close\")"
            n92 = Unbundle By Name(w267) -> ("Core.Current VI Reference"=w266:refnum<vi>)
            n93 = disable-structure shown="Default" {
              disable-tunnel: w269 -> [w275 w298]
              disable-tunnel: [w274 w298] -> w268
              disable-tunnel: w266 -> [w273 _]
              disable-tunnel: w265 -> [w272 _]
              frame condition #0 (active) {
                n94 = case shown="\"Close\"" w272 {
                  tunnel: w275 -> [w279 w292]
                  tunnel: [w281 w293] -> w274
                  tunnel: w273 -> [w280 w290]
                  frame "Open", Default {
                    n95 = property class="VI"(reference=w280, error in=w279) -> (reference out=w277:refnum<vi>, error out=w278:errorcluster, "FP.State"=w276:T3)
                    n96 = case shown="\"Closed\"" w276 {
                      tunnel: [w284 w287] -> w281
                      tunnel: w278 -> [w283 w287]
                      tunnel: w277 -> [w282 _]
                      frame "Closed" {
                        n97 = invoke class="VI" method="FP.Open"(reference=w282, error in=w283, "Activate"=TRUE, "State"=T3."Standard") -> (error out=w284:errorcluster)  [unwired: 1 in, 4 out]
                      }
                      frame Default {
                      }
                    }
                  }
                  frame "Close" {
                    n98 = property class="VI"(reference=w290, error in=w292) -> (reference out=w289:refnum<vi>, error out=w291:errorcluster, "FP.State"=w288:T3)
                    n99 = case shown="Default" w288 {
                      tunnel: [w294 w297] -> w293
                      tunnel: w291 -> [w294 w296]
                      tunnel: w289 -> [_ w295]
                      frame "Invalid", "Closed" {
                      }
                      frame Default {
                        n100 = invoke class="VI" method="FP.Close"(reference=w295, error in=w296) -> (error out=w297:errorcluster)  [unwired: 1 in, 2 out]
                      }
                    }
                  }
                }
              }
              frame condition #1 {
              }
            }
            n101 = call <vilib>:"Add State(s) to Queue__jki_lib_state_machine.vi"("State(s) in (\"\")"=w271) -> ("States Out"=w270:string)  [unwired: 14 in]
          }
          frame "---------- Macro ----------" {
            # "Do not put any code in this frame.\n(It is a separator no-op. You can make a copy of this frame to create a new Macro frame)"
            n102 = call <vilib>:"Add State(s) to Queue__jki_lib_state_machine.vi"("State(s) in (\"\")"=w303) -> ("States Out"=w302:string)  [unwired: 14 in]
          }
          frame "Macro: Initialize" {
            w306 = "UI: Initialize\n//UI: Front Panel State >> Open"  # UI: Initialize //UI: Front Panel State >> Open
            # "Initialization Macro\n(This is called once, when the VI starts)"
            n103 = call <vilib>:"Add State(s) to Queue__jki_lib_state_machine.vi"("State(s) in Front (\"\")"="Data: Initialize\nInitialize Core Data\nEvents: Register", "State(s) in (\"\")"="Process: Sync", "State(s) at Back (\"\")"=w306) -> ("States Out"=w305:string)  [unwired: 12 in]
            n104 = call <vilib>:"Add State(s) to Queue__jki_lib_state_machine.vi"("State(s) in Front (\"\")"=w305, "State(s) in (\"\")"=w312) -> ("States Out"=w311:string)  [unwired: 13 in]
          }
          frame "Macro: Exit" {
            # "Exit Macro\n(This is called once, when the VI exits)"
            n105 = Unbundle By Name(w317) -> ("Core.Close Panel on Exit?"=w323:bool)
            n106 = Select(t="//UI: Front Panel State >> Close", s=w323, f="") -> (s? t:f=w320:string)
            n107 = call <vilib>:"Add State(s) to Queue__jki_lib_state_machine.vi"("State(s) in Front (\"\")"="Data: Cleanup\nEvents: Unregister", "State(s) in (\"\")"="Process: Sync", "State(s) at Back (\"\")"="Exit") -> ("States Out"=w314:string)  [unwired: 12 in]
            n108 = call <vilib>:"Add State(s) to Queue__jki_lib_state_machine.vi"("State(s) in (\"\")"=w320, "State(s) at Back (\"\")"=w314) -> ("States Out"=w319:string)  [unwired: 13 in]
            n109 = call <vilib>:"Add State(s) to Queue__jki_lib_state_machine.vi"("State(s) in Front (\"\")"=w319, "State(s) in (\"\")"=w326) -> ("States Out"=w325:string)  [unwired: 13 in]
          }
          frame "---------- Process ----------" {
            # "Template Separator\n(You can make a copy of, or modify, this frame)"
            n110 = call <vilib>:"Add State(s) to Queue__jki_lib_state_machine.vi"("State(s) in (\"\")"=w331) -> ("States Out"=w330:string)  [unwired: 14 in]
          }
          frame "Process: Sync" {
            n111 = Unbundle By Name(w339) -> ("Self Reference"=w335:refnum<class "DisplayWaveforms.lvclass">)
            n112 = call <vilib>:"WaitOnProcessSync.vi"("error in (no error)"=w334, "SMO"=w335) -> ("error out"=w333:errorcluster, "Don't run?"=w338:bool)  [unwired: 7 in, 1 out]
            n113 = Select(t="Data: Cleanup\nEvents: Unregister\nExit", s=w338, f="") -> (s? t:f=w332:string)
            n114 = call <vilib>:"Add State(s) to Queue__jki_lib_state_machine.vi"("State(s) in Front (\"\")"=w332, "State(s) in (\"\")"=w342) -> ("States Out"=w341:string)  [unwired: 13 in]
          }
          frame "---------- Events ----------" {
            # "Template Separator\n(You can make a copy of, or modify, this frame)"
            n115 = call <vilib>:"Add State(s) to Queue__jki_lib_state_machine.vi"("State(s) in (\"\")"=w347) -> ("States Out"=w346:string)  [unwired: 14 in]
          }
          frame "Events: Register" {
            w354 = cluster{"New Value":refnum<user-event>} {"New Value"=refnum}  # Dependency.PublicEvents
            # "Get Event from SMO"
            # "Register for Data Producer Event here..."
            n116 = Unbundle By Name(w363) -> ("Self Reference"=w357:refnum<class "DisplayWaveforms.lvclass">)
            n117 = call <vilib>:"GetProtectedEvents.vi"("SMO"=w357) -> ("error out"=w352:errorcluster, "SMO Protected Events"=w361:T11)  [unwired: 8 in, 1 out]
            n118 = call "Chart[Template].GetProtectedEvents.vi"("DisplayWaveforms"=w357) -> ("error out"=w353:errorcluster, "Protected Events"=w358:T12)  [unwired: 8 in, 1 out]
            n119 = call "Chart[Template].GetDependencies.vi"("DisplayWaveforms"=w357) -> ("error out"=w351:errorcluster, "Dependencies"=w355:T13)  [unwired: 8 in, 1 out]
            n120 = Unbundle By Name(w355) -> ("New Value"=w350:refnum<user-event>)
            n121 = Not A Number/Path/Refnum?(number/path/refnum=w350) -> (NaN/Path/Refnum?=w349:bool)
            n122 = case shown="False" w349 {
              tunnel: w350 -> [w366 _]
              tunnel: w354 -> [w368 w371]
              tunnel: [w367 w370] -> w348
              frame False {
                n123 = Bundle By Name(cluster=w368, "New Value"=w366) -> (w367:cluster{"New Value":refnum<user-event>})
              }
              frame True {
                n124 = Bundle By Name(cluster=w371, "New Value"=refnum<user-event> refnum) -> (w370:cluster{"New Value":refnum<user-event>})
              }
            }
            n125 = register-events(w361, w358, w348) -> (reference out=w362:refnum<event-registration>, error out=w359:errorcluster)  [unwired: 2 in]
            n126 = Merge Errors(w356, w359, w351, w352, w353) -> (w360:errorcluster)
            n127 = call <vilib>:"Add State(s) to Queue__jki_lib_state_machine.vi"("State(s) in (\"\")"=w365) -> ("States Out"=w364:string)  [unwired: 14 in]
          }
          frame "Events: Unregister" {
            n128 = Unregister For Events(event registration refnum=w374, error in=w373) -> (error out=w372:errorcluster)
            n129 = call <vilib>:"Clear Errors.vi"("error in (no error)"=w372) -> ()  [unwired: 5 in, 2 out]
            n130 = call <vilib>:"Add State(s) to Queue__jki_lib_state_machine.vi"("State(s) in (\"\")"=w377) -> ("States Out"=w376:string)  [unwired: 14 in]
          }
          frame "---------- Action ----------" {
            n131 = call <vilib>:"Add State(s) to Queue__jki_lib_state_machine.vi"("State(s) in (\"\")"=w382) -> ("States Out"=w381:string)  [unwired: 14 in]
          }
          frame "Action: Clear Chart" {
            n132 = Unbundle By Name(w386) -> ("Self Reference"=w383:refnum<class "DisplayWaveforms.lvclass">)
            n133 = call-dynamic "Chart[Template].Clear.vi"("error in (no error)"=w385, "DisplayWaveforms"=w383) -> ("error out"=w384:errorcluster)  [unwired: 8 in, 1 out]
            n134 = call <vilib>:"Add State(s) to Queue__jki_lib_state_machine.vi"("State(s) in (\"\")"=w389) -> ("States Out"=w388:string)  [unwired: 14 in]
          }
          frame "Action: Export Chart" {
            # "Save snapshot of front panel"
            n135 = Unbundle By Name(w402) -> ("Self Reference"=w400:refnum<class "DisplayWaveforms.lvclass">, "Export Folder Path"=w394:path)
            n136 = call-dynamic "Chart[Template].Export.vi"("error in (no error)"=w401, "Export Folder Path"=w394, "DisplayWaveforms"=w400) -> ("error out"=w397:errorcluster)  [unwired: 7 in, 1 out]
            n137 = control-ref of="This VI"() -> (w390:refnum<vi>)
            n138 = invoke class="VI" method="FP.Get Image"(reference=w390, error in=w397, "visible area only"=TRUE ("Visible Area Only"), "image depth"=0 ("Image Depth")) -> (error out=w393:errorcluster, "image data"=w396:T14)  [unwired: 2 in, 4 out]
            n139 = Build Path(base path=w394, name or relative path=path "all_charts.png") -> (appended path=w395:path)
            n140 = call <vilib>:"Write PNG File.vi"("error in (no error)"=w393, "image data"=w396, "path to PNG file"=w395) -> ("error out"=w392:errorcluster)  [unwired: 7 in, 1 out]
            n141 = disable-structure shown="Disabled" {
              disable-tunnel: w390 -> [w406 _]
              frame Disabled {
                # "Enable to print to pdf for \nbetter quality for thesis."
                n142 = invoke class="VI" method="Print.Panel To Printer"(reference=w406) -> ()  [unwired: 3 in, 4 out]
              }
              frame Enabled {
              }
            }
            n143 = call <vilib>:"Add State(s) to Queue__jki_lib_state_machine.vi"("State(s) in (\"\")"=w405) -> ("States Out"=w404:string)  [unwired: 14 in]
          }
          frame "Action: SetChartParams" {
            n144 = Unbundle By Name(w411) -> ("Self Reference"=w408:refnum<class "DisplayWaveforms.lvclass">, "ChartParams"=w407:T4)
            n145 = call-dynamic "Chart[Template].SetParams.vi"("error in (no error)"=w410, "ChartParams"=w407, "DisplayWaveforms"=w408) -> ("error out"=w409:errorcluster)  [unwired: 7 in, 1 out]
            n146 = call <vilib>:"Add State(s) to Queue__jki_lib_state_machine.vi"("State(s) in (\"\")"=w414) -> ("States Out"=w413:string)  [unwired: 14 in]
          }
          frame "Action: Notify UI Closed" {
            # "Notify that the UI has been closed"
            n147 = Unbundle By Name(w417) -> ("Self Reference"=w418:refnum<class "DisplayWaveforms.lvclass">)
            n148 = call <vilib>:"Hide.vi"("error in (no error)"=w416, "SMO.UI"=w418) -> ("error out"=w415:errorcluster)  [unwired: 8 in, 1 out]
            n149 = call <vilib>:"Add State(s) to Queue__jki_lib_state_machine.vi"("State(s) in (\"\")"=w421) -> ("States Out"=w420:string)  [unwired: 14 in]
          }
        }
      }
    }
    frame Error {
    }
  }
  n150 = call-parent "Process.vi"("error in (no error)"=w8, "SMO.UI"=w7) -> ("error out"=w5:errorcluster, "SMO.UI out"=→"DisplayWaveforms out":refnum<class "DisplayWaveforms.lvclass">)  [unwired: 8 in]
  n151 = Merge Errors(w5, w4) -> (→"error out":errorcluster)
